vi "lumencor_on.vi"   [LabVIEW 2011]
uses:
  <vilib>/DAQmx/write.llb/DAQmx Write.vi
  <vilib>/DAQmx/write.llb/DAQmx Write (Analog 1D DBL NChan 1Samp).vi
  <vilib>/DAQmx/miscellaneous.llb/DAQmx Fill In Error Info.vi
types:
  T1 = enum32{"Invalid", "Standard", "Closed", "Hidden", "Minimized", "Maximized"}
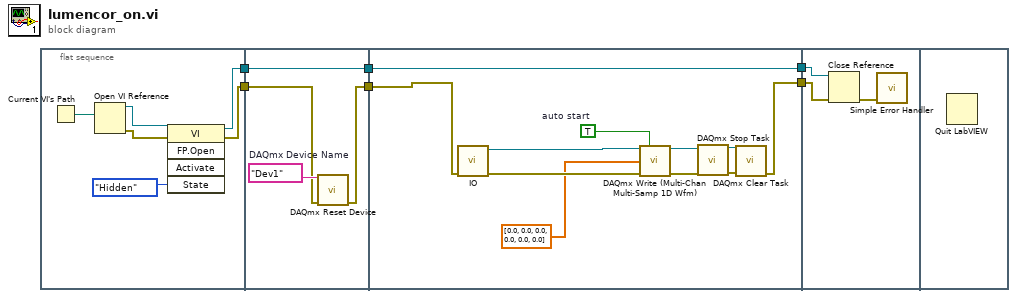
[diagram p0: block diagram]
diagram:
  n1 = flat-sequence {
    tunnel: [w8] -> w4
    tunnel: [w7] -> w2
    tunnel: w4 -> [w16]
    tunnel: [w16] -> w3
    tunnel: w2 -> [w14]
    tunnel: [w13] -> w1
    tunnel: [w23] -> w6
    tunnel: w3 -> [w23]
    tunnel: w1 -> [w22]
    tunnel: [w17] -> w5
    tunnel: w6 -> [w30]
    tunnel: w5 -> [w29]
    frame #0 {
      n2 = Current VI's Path() -> (path=w9:path)
      n3 = Open VI Reference(vi path=w9) -> (vi reference=w10:refnum<vi>, error out=w11:errorcluster)  [unwired: 5 in]
      n4 = invoke class="VI" method="FP.Open"(reference=w10, error in=w11, "State"=T1."Hidden") -> (reference out=w8:refnum<vi>, error out=w7:errorcluster)  [unwired: 2 in, 3 out]
    }
    frame #1 {
      w15 = tag "Dev1"  # DAQmx Device Name
      n5 = call <vilib>:"DAQmx Reset Device.vi"("device in"=w15, "error in"=w14) -> ("error out"=w13:errorcluster)  [unwired: 13 in]
    }
    frame #2 {
      w27 = TRUE  # auto start
      n6 = call "IO.vi"("error in"=w22) -> ("error out"=w25:errorcluster, "task out"=w26:refnum<k21>)  [unwired: 9 in]
      n7 = call-poly "DAQmx Write (Multi-Chan Multi-Samp 1D Wfm).vi"("task/channels in"=w26, "auto start"=w27, "data"=dbl[] [0.0, 0.0, 0.0, 0.0, 0.0, 0.0], "error in"=w25) -> ("task out"=w21:refnum<k21>, "error out"=w20:errorcluster)  [unwired: 10 out]
      n8 = call <vilib>:"DAQmx Stop Task.vi"("task/channels in"=w21, "error in"=w20) -> ("task out"=w19:refnum<k21>, "error out"=w18:errorcluster)  [unwired: 12 in]
      n9 = call <vilib>:"DAQmx Clear Task.vi"("task in"=w19, "error in"=w18) -> ("error out"=w17:errorcluster)  [unwired: 13 in]
    }
    frame #3 {
      n10 = Close Reference(reference=w30, error in (no error)=w29) -> (error out=w28:errorcluster)
      n11 = call <vilib>:"Simple Error Handler.vi"("error in (no error)"=w28) -> ()  [unwired: 4 in, 5 out]
    }
    frame #4 {
      n12 = Quit LabVIEW() -> ()  [unwired: 1 in]
    }
  }
